vi "Vaisala Server.vi"(11 "DVR In":refnum<data-value>) -> (3 "DVR Out":refnum<data-value>)   [LabVIEW 2016]
uses:
  Data/Nicholas Data.lvclass
  Session/Raw FPGA/FPGA Session.lvclass
  C:/Program Files (x86)/National Instruments/LabVIEW 2016/vi.lib/MSR Consulting, LLC/General Reuse/Session APIs/_Session Fwk/Session - Root.lvclass
  <vilib>/MSR Consulting, LLC/General Reuse/Session APIs/Session Log/System Log.lvclass
  <vilib>/MSR Consulting, LLC/General Reuse/Session APIs/File Access/Config Data/Config Data.lvclass
  Session/Session/FPGA Serial.lvclass
  C:/Program Files (x86)/National Instruments/LabVIEW 2016/vi.lib/MSR Consulting, LLC/General Reuse/Session APIs/Serial/Serial Session.lvclass
  <vilib>/MSR Consulting, LLC/General Reuse/Data/Array Data/Single 1-D/Single_Array.lvclass
  <vilib>/MSR Consulting, LLC/General Reuse/Session APIs/Session Log/System Log.lvclass/System Log.ctl
  <vilib>/MSR Consulting, LLC/General Reuse/Session APIs/File Access/Config Data/Config Data.lvclass/Config Data.ctl
  <vilib>/MSR Consulting, LLC/Devices/Vaisala/Vaisala.lvclass
  C:/Program Files (x86)/National Instruments/LabVIEW 2016/vi.lib/MSR Consulting, LLC/Devices/Configurable Device/Configurable Device.lvclass
  <vilib>/MSR Consulting, LLC/Devices/Configurable Device/Configurable Device.lvclass/Configurable Device.ctl
  Session/Session/FPGA Serial.lvclass/FPGA Serial.ctl
  <vilib>/MSR Consulting, LLC/General Reuse/Session APIs/Serial/Serial Session.lvclass/Serial Session.ctl
  <vilib>/MSR Consulting, LLC/Devices/Vaisala/Vaisala.lvclass/Vaisala.ctl
  Data/Nicholas Data.lvclass/Nicholas Data.ctl
  <vilib>/MSR Consulting, LLC/Devices/Configurable Device/Write ID.vi
  Session/Session/Write FPGA Session.vi
  <vilib>/MSR Consulting, LLC/General Reuse/Session APIs/Serial/Public/Accessors/Write Sys Log.vi
  <vilib>/MSR Consulting, LLC/Devices/Configurable Device/Write Handle.vi
  <vilib>/MSR Consulting, LLC/Devices/Vaisala/Accessors/Write hSession.vi
  Data/Write Vaisala Data.vi
  <vilib>/MSR Consulting, LLC/General Reuse/Session APIs/File Access/Config Data/Accessors/Write Cfg Path.vi
  <vilib>/MSR Consulting, LLC/General Reuse/Session APIs/Session Log/Accessors/Write Main Path.vi
  <vilib>/MSR Consulting, LLC/General Reuse/Session APIs/_Session Fwk/Session - Root.lvclass
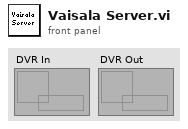
[diagram p1: front panel]
types:
  T1 = typedef "Session - Root.lvclass/Session Handle.ctl" = refnum<data-value>
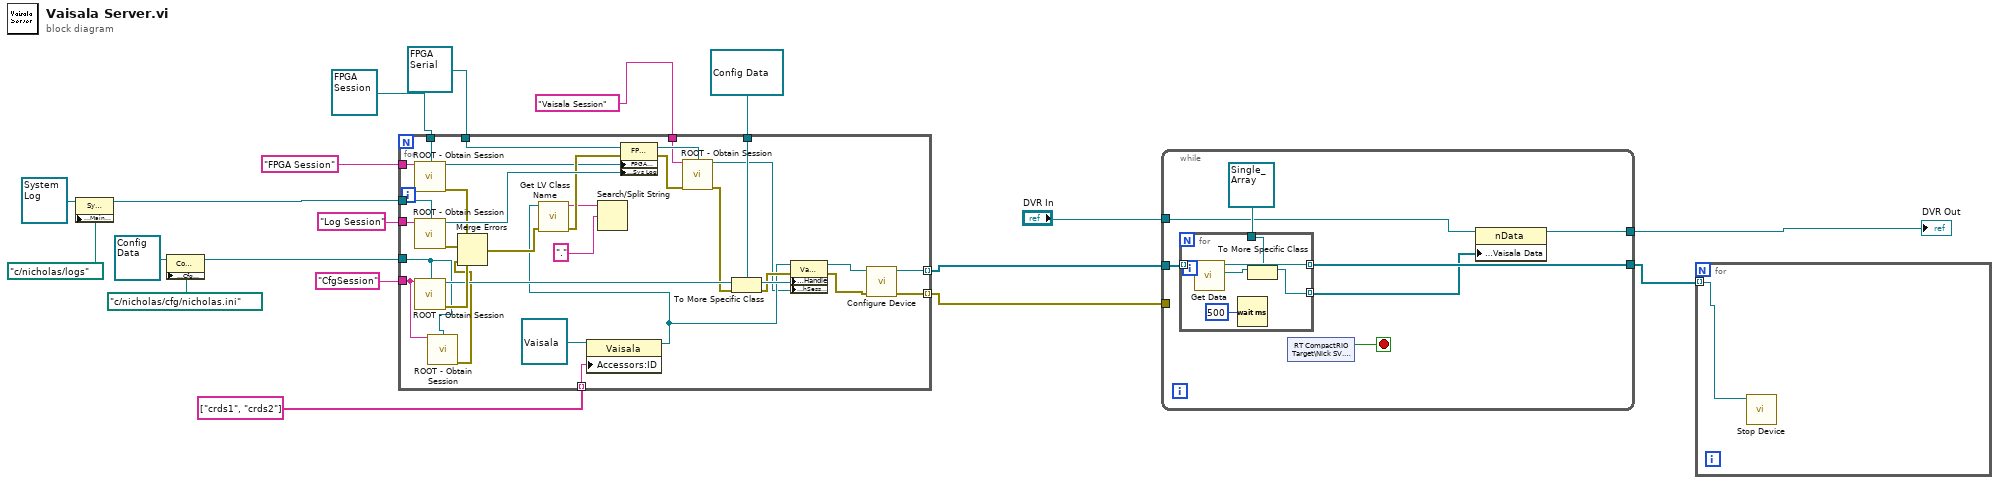
[diagram p0: block diagram]
diagram:
  n1 = property class="Sys Log"(reference=refnum<class "System Log.lvclass"> refnum ("Sys Log"), "Accessors:Main Path"=path "c:/nicholas/logs" ("Main Path")) -> (reference out=w10:refnum<class "System Log.lvclass">)  [unwired: 1 in, 1 out]
  n2 = property class="Config Data"(reference=refnum<class "Config Data.lvclass"> refnum ("Config Data"), "Accessors:Cfg Path"=path "c:/nicholas/cfg/nicholas.ini" ("Cfg Path")) -> (reference out=w11:refnum<class "Config Data.lvclass">)  [unwired: 1 in, 1 out]
  n3 = for {
    tunnel: w10 -> [w52]
    tunnel: "Log Session" ("Session Name ()") -> [w51]
    tunnel: refnum<class "FPGA Session.lvclass"> refnum ("FPGA Session") -> [w50]
    tunnel: "FPGA Session" ("Session Name ()") -> [w49]
    tunnel: w11 -> [w30]
    tunnel: "CfgSession" ("Session Name ()") -> [w31]
    tunnel: refnum<class "FPGA Serial.lvclass"> refnum ("FPGA Serial.lvclass") -> [w48]
    tunnel: refnum<data-value> refnum ("Session Handle") -> [w37]
    tunnel: "Vaisala Session" ("Session Name ()") -> [w32]
    tunnel: string[] ["crds1", "crds2"] -> [w25] mode=indexing
    tunnel: [w22] -> w8 mode=indexing
    tunnel: [w21] -> w4 mode=indexing
    n4 = call <vilib>:"ROOT - Obtain Session.vi"("Session Name ()"=w49, "OBJ - Session"=w50) -> ("Session Handle"=w20:T1, "error out"=w45:errorcluster)  [unwired: 11 in, 1 out]
    n5 = call <vilib>:"ROOT - Obtain Session.vi"("Session Name ()"=w51, "OBJ - Session"=w52) -> ("Session Handle"=w46:T1, "error out"=w44:errorcluster)  [unwired: 11 in, 1 out]
    n6 = call <vilib>:"ROOT - Obtain Session.vi"("Session Name ()"=w31, "OBJ - Session"=w30) -> ("Session Handle"=w41:T1, "error out"=w43:errorcluster)  [unwired: 11 in, 1 out]
    n7 = call <vilib>:"ROOT - Obtain Session.vi"("Session Name ()"=w31, "OBJ - Session"=w30) -> ("error out"=w29:errorcluster)  [unwired: 11 in, 2 out]
    n8 = Merge Errors(w45, w44, w43, w29) -> (w36:errorcluster)
    n9 = property class="Vaisala"(reference=refnum<class "Vaisala.lvclass"> refnum ("Vaisala"), "Accessors:ID"=w25) -> (reference out=w27:refnum<class "Vaisala.lvclass">)  [unwired: 1 in, 1 out]
    n10 = call <vilib>:"Get LV Class Name.vi"("error in (no error)"=w36, "object"=w27) -> ("error out"=w35:errorcluster, "class name"=w33:string)  [unwired: 8 in]
    n11 = Search/Split String(string=w33, search string/char (-)="." ("regular expression")) -> ()  [unwired: 1 in, 3 out]
    n12 = property class="FPGA Serial.lvclass"(reference=w48, error in=w35, "FPGA Session"=w20, "Public:Accessors:Sys Log"=w46) -> (reference out=w47:refnum<class "FPGA Serial.lvclass">, error out=w42:errorcluster)
    n13 = call <vilib>:"ROOT - Obtain Session.vi"("Session Name ()"=w32, "OBJ - Session"=w47, "error in (no error)"=w42) -> ("Session Handle"=w26:T1, "error out"=w39:errorcluster)  [unwired: 10 in, 1 out]
    n14 = To More Specific Class(target class=w37, reference=w41, error in=w39) -> (specific class reference=w40:refnum<data-value>, error out=w38:errorcluster)
    n15 = property class="Vaisala"(reference=w27, error in=w38, "Accessors:Handle"=w40, "Accessors:hSession"=w26) -> (reference out=w24:refnum<class "Vaisala.lvclass">, error out=w23:errorcluster)
    n16 = call-dynamic "Configure Device.vi"("error in"=w23, "Vaisala Probe in"=w24) -> ("error out"=w21:errorcluster, "Vaisala Probe out"=w22:refnum<class "Vaisala.lvclass">)  [unwired: 6 in, 2 out]
  }
  n17 = while {
    tunnel: w8 -> [w59]
    tunnel: [w58] -> w3
    tunnel: "DVR In" -> [w55]
    tunnel: [w54] -> w6
    tunnel: w4 -> [_]
    stop <- w57 stop-if-true
    n18 = for {
      tunnel: w59 -> [w65] mode=indexing
      tunnel: [w64] -> w58 mode=indexing
      tunnel: refnum<class "Single_Array.lvclass"> refnum ("Base Data Lib:[SGL]") -> [w62]
      tunnel: [w61] -> w53 mode=indexing
      n19 = call-dynamic "Get Data.vi"("Cfg Dev in"=w65) -> ("Data"=w63:refnum<class "Data.lvclass">, "Cfg Dev out"=w64:refnum<class "Vaisala.lvclass">)  [unwired: 8 in, 1 out]
      n20 = Wait (ms)(milliseconds to wait=u32 500) -> ()  [unwired: 1 out]
      n21 = To More Specific Class(target class=w62, reference=w63) -> (specific class reference=w61:refnum<class "Single_Array.lvclass">)  [unwired: 1 in, 1 out]
    }
    n22 = shared-variable "RT CompactRIO Target\\Nick SV.lvlib\\Stop"() -> (w57:bool)  [unwired: 1 in, 1 out]
    n23 = property class="nData"(reference=w55, "Accessors:Vaisala Data"=w53) -> (reference out=w54:refnum<data-value>)  [unwired: 1 in, 1 out]
  }
  "DVR Out" <- w6
  n24 = for {
    tunnel: w3 -> [w66] mode=indexing
    n25 = call-dynamic "Stop Device.vi"("Cfg Dev in"=w66) -> ()  [unwired: 9 in, 2 out]
  }
